vi "Func-엑셀 데이터를 그래프로 출력.vi"() -> ()   [LabVIEW 2015] (continued)
57.566\n45\t44.56\t57.56\n45\t44.56\t57.556\n45\t44.56\t57.547\n45\t44.56\t57.539\n45\t44.57\t57.535\n45\t44.57\t57.527\n45\t44.57\t57.522\n45\t44.58\t57.516\n45\t44.58\t57.513\n45\t44.58\t57.505\n45\t44.59\t57.495\n45\t44.59\t57.484\n45\t44.59\t57.475\n45\t44.59\t57.464\n45\t44.59\t57.451\n45\t44.6\t57.446\n45\t44.6\t57.445\n45\t44.6\t57.439\n45\t44.6\t57.435\n45\t44.61\t57.427\n45\t44.61\t57.424\n45\t44.61\t57.42\n45\t44.62\t57.407\n45\t44.62\t57.401\n45\t44.62\t57.397\n45\t44.62\t57.388\n45\t44.62\t57.386\n45\t44.63\t57.376\n45\t44.63\t57.366\n45\t44.64\t57.362\n45\t44.64\t57.358\n45\t44.64\t57.348\n45\t44.64\t57.339\n45\t44.64\t57.333\n45\t44.64\t57.33\n45\t44.64\t57.324\n45\t44.64\t57.311\n45\t44.65\t57.306\n45\t44.65\t57.302\n45\t44.66\t57.299\n45\t44.66\t57.284\n45\t44.67\t57.276\n45\t44.67\t57.272\n45\t44.67\t57.264\n45\t44.67\t57.255\n45\t44.68\t57.244\n45\t44.68\t57.24\n45\t44.68\t57.232\n45\t44.69\t57.225\n45\t44.69\t57.22\n45\t44.69\t57.216\n45\t44.7\t57.209\n45\t44.7\t57.203\n45\t44.7\t57.199\n45\t44.71\t57.189\n45\t44.71\t57.184\n45\t44.71\t57.18\n45\t44.71\t57.178\n45\t44.71\t57.173\n45\t44.72\t57.169\n45\t44.72\t57.159\n45\t44.73\t57.15\n45\t44.73\t57.139\n45\t44.73\t57.128\n45\t44.73\t57.12\n45\t44.73\t57.112\n45\t44.73\t57.105\n45\t44.73\t57.101\n45\t44.73\t57.097\n45\t44.74\t57.093\n45\t44.74\t57.086\n45\t44.74\t57.078\n45\t44.74\t57.073\n45\t44.75\t57.063\n45\t44.75\t57.056\n45\t44.75\t57.051\n45\t44.76\t57.048\n45\t44.76\t57.042\n45\t44.76\t57.037\n45\t44.77\t57.034\n45\t44.77\t57.025\n45\t44.77\t57.018\n45\t44.77\t57.013\n45\t44.77\t57.004\n45\t44.78\t56.999\n45\t44.78\t56.995\n45\t44.78\t56.989\n45\t44.78\t56.982\n45\t44.79\t56.973\n45\t44.8\t56.964\n45\t44.8\t56.957\n45\t44.8\t56.951\n45\t44.8\t56.937\n45\t44.8\t56.932\n45\t44.8\t56.927\n45\t44.8\t56.923\n45\t44.81\t56.917\n45\t44.81\t56.909\n45\t44.81\t56.902\n45\t44.81\t56.896\n45\t44.81\t56.886\n45\t44.81\t56.883\n45\t44.82\t56.88\n45\t44.82\t56.87\n45\t44.82\t56.866\n45\t44.82\t56.86\n45\t44.82\t56.854\n45\t44.82\t56.845\n45\t44.82\t56.835\n45\t44.82\t56.832\n45\t44.83\t56.829\n45\t44.83\t56.824\n45\t44.83\t56.816\n45\t44.83\t56.81\n45\t44.83\t56.807\n45\t44.83\t56.798\n45\t44.83\t56.794\n45\t44.83\t56.787\n45\t44.83\t56.784\n45\t44.83\t56.78\n45\t44.84\t56.772\n45\t44.84\t56.769\n45\t44.83\t56.761\n45\t44.84\t56.754\n45\t44.84\t56.744\n45\t44.84\t56.738\n45\t44.84\t56.735\n45\t44.84\t56.725\n45\t44.84\t56.724\n45\t44.84\t56.724\n45\t44.84\t56.716\n45\t44.85\t56.711\n45\t44.86\t56.698\n45\t44.87\t56.699\n45\t44.88\t56.693\n45\t44.89\t56.681\n45\t44.9\t56.676\n45\t44.91\t56.669\n45\t44.92\t56.659\n45\t44.93\t56.65\n45\t44.94\t56.642\n45\t44.95\t56.632\n45\t44.96\t56.629\n45\t44.97\t56.626\n45\t44.98\t56.623\n45\t45\t56.616\n45\t44.96\t56.611\n45\t44.96\t56.606\n45\t44.96\t56.6\n45\t44.96\t56.593\n45\t44.96\t56.581\n45\t44.96\t56.576\n45\t44.96\t56.566\n45\t44.96\t56.561\n45\t44.96\t56.555\n45\t44.96\t56.548\n45\t44.96\t56.547\n45\t44.96\t56.542\n45\t44.96\t56.539\n45\t44.96\t56.531\n45\t44.96\t56.526\n45\t44.96\t56.519\n45\t44.96\t56.513\n45\t44.96\t56.51\n45\t44.96\t56.502\n45\t44.96\t56.5\n45\t44.96\t56.493\n45\t44.96\t56.485\n45\t44.97\t56.48\n45\t44.97\t56.47\n45\t44.97\t56.461\n45\t44.97\t56.455\n45\t44.97\t56.449\n45\t44.97\t56.444\n45\t44.97\t56.437\n45\t44.97\t56.435\n45\t44.97\t56.428\n45\t44.97\t56.423\n45\t44.97\t56.418\n45\t44.97\t56.412\n45\t44.97\t56.411\n45\t44.97\t56.403\n45\t44.97\t56.399\n45\t44.97\t56.389\n45\t44.97\t56.383\n45\t44.97\t56.38\n45\t44.97\t56.372\n45\t44.97\t56.367\n45\t44.97\t56.362\n45\t44.97\t56.36\n45\t44.97\t56.353\n45\t44.97\t56.345\n45\t44.97\t56.34\n45\t44.97\t56.333\n45\t44.97\t56.327\n45\t44.97\t56.323\n45\t44.97\t56.317\n45\t44.97\t56.311\n45\t44.97\t56.304\n45\t44.97\t56.297\n45\t44.97\t56.291\n45\t44.97\t56.286\n45\t44.98\t56.278\n45\t44.98\t56.276\n45\t44.97\t56.275\n45\t44.97\t56.268\n45\t44.97\t56.264\n45\t44.97\t56.261\n45\t44.98\t56.26\n45\t44.98\t56.256\n45\t44.98\t56.25\n45\t44.98\t56.243\n45\t44.98\t56.239\n45\t44.98\t56.227\n45\t44.98\t56.216\n45\t44.98\t56.207\n45\t44.98\t56.203\n45\t44.98\t56.198\n45\t44.98\t56.192\n45\t44.98\t56.183\n45\t44.98\t56.18\n45\t44.98\t56.175\n45\t44.98\t56.167\n45\t44.98\t56.161\n45\t44.98\t56.16\n45\t44.98\t56.156\n45\t44.98\t56.154\n45\t44.98\t56.147\n45\t44.98\t56.138\n45\t44.98\t56.136\n45\t44.98\t56.125\n45\t44.98\t56.121\n45\t44.98\t56.113\n45\t44.98\t56.107\n45\t44.98\t56.104\n45\t44.98\t56.101\n45\t44.98\t56.092\n45\t44.98\t56.088\n45\t44.98\t56.082\n45\t44.98\t56.08\n45\t44.98\t56.076\n45\t44.98\t56.068\n45\t44.98\t56.066\n45\t44.98\t56.06\n45\t44.98\t56.06\n45\t44.98\t56.055\n45\t44.98\t56.047\n45\t44.98\t56.045\n45\t44.98\t56.035\n45\t44.98\t56.031\n45\t44.98\t56.025\n45\t44.98\t56.019\n45\t44.98\t56.018\n45\t44.98\t56.015\n45\t44.98\t56.007\n45\t45\t56.003\n45\t45\t55.997\n45\t45\t55.987\n45\t45\t55.978\n45\t45\t55.97\n45\t45\t55.969\n45\t45\t55.966\n45\t45\t55.962\n45\t45\t55.956\n45\t45\t55.954\n45\t45\t55.944\n45\t45\t55.941\n45\t45\t55.932\n45\t45\t55.924\n45\t45\t55.92\n45\t45\t55.916\n45\t45\t55.912\n45\t45\t55.907\n45\t45\t55.903\n45\t45\t55.895\n45\t45\t55.89\n45\t45\t55.884\n45\t44.98\t55.875\n45\t44.98\t55.868\n45\t45\t55.866\n45\t45\t55.862\n45\t45\t55.86\n45\t45\t55.857\n45\t44.98\t55.85\n45\t44.98\t55.849\n45\t44.98\t55.842\n45\t44.98\t55.834\n45\t44.98\t55.828\n45\t44.98\t55.823\n45\t44.98\t55.817\n45\t44.98\t55.811\n45\t44.98\t55.805\n45\t44.98\t55.801\n45\t44.98\t55.797\n45\t44.98\t55.787\n45\t44.98\t55.787\n45\t44.98\t55.782\n45\t44.98\t55.777\n45\t44.98\t55.772\n45\t44.98\t55.768\n45\t44.98\t55.762\n45\t44.98\t55.758\n45\t44.98\t55.755\n45\t44.98\t55.75\n45\t44.98\t55.745\n45\t44.98\t55.742\n45\t44.98\t55.736\n45\t44.98\t55.731\n45\t44.98\t55.727\n45\t44.98\t55.727\n45\t44.98\t55.72\n45\t44.98\t55.716\n45\t44.98\t55.713\n45\t45\t55.708\n45\t45\t55.698\n45\t44.98\t55.693\n45\t44.98\t55.69\n45\t45\t55.682\n45\t45\t55.681\n45\t45\t55.675\n45\t45\t55.671\n45\t45\t55.664\n45\t45\t55.661\n45\t45\t55.659\n45\t45\t55.652\n45\t45\t55.649\n45\t45\t55.643\n45\t45\t55.639\n45\t45\t55.631\n45\t45\t55.621\n45\t45\t55.618\n45\t45\t55.61\n45\t45\t55.607\n45\t45\t55.604\n45\t45\t55.602\n45\t45\t55.597\n45\t45\t55.589\n45\t45\t55.587\n45\t45\t55.581\n45\t45\t55.576\n45\t45\t55.575\n45\t45\t55.573\n45\t45\t55.571\n45\t45\t55.569\n45\t45\t55.557\n45\t45\t55.553\n45\t45\t55.543\n45\t45\t55.534\n45\t45\t55.53\n45\t45\t55.523\n45\t45\t55.521\n45\t45\t55.518\n45\t45\t55.511\n45\t45\t55.508\n45\t45\t55.502\n45\t45\t55.498\n45\t45\t55.494\n45\t45\t55.489\n45\t45\t55.486\n45\t45\t55.48\n45\t45\t55.475\n45\t45\t55.465\n45\t45\t55.46\n45\t45\t55.455\n45\t45\t55.449\n45\t45\t55.448\n45\t45\t55.445\n45\t45\t55.439\n45\t45\t55.436\n45\t45\t55.435\n45\t45\t55.429\n45\t45\t55.425\n45\t45\t55.42\n45\t45\t55.418\n45\t45\t55.416\n45\t45\t55.411\n45\t45\t55.406\n45\t45\t55.401\n45\t45\t55.391\n45\t45\t55.386\n45\t45\t55.381\n45\t45\t55.369\n45\t45\t55.368\n45\t45\t55.365\n45\t45\t55.365\n45\t45\t55.362\n45\t45\t55.357\n45\t45\t55.359\n45\t45\t55.354\n45\t45\t55.348\n45\t45\t55.344\n45\t45\t55.339\n45\t45\t55.333\n45\t45\t55.325\n45\t45\t55.323\n45\t45\t55.319\n45\t44.98\t55.312\n45\t44.98\t55.312\n45\t44.98\t55.309\n45\t44.98\t55.307\n45\t44.98\t55.299\n45\t44.98\t55.292\n45\t44.98\t55.287\n45\t44.98\t55.281\n45\t45\t55.277\n45\t45\t55.271\n45\t45\t55.268\n45\t44.98\t55.264\n45\t44.98\t55.259\n45\t44.98\t55.256\n45\t44.98\t55.247\n45\t44.98\t55.243\n45\t44.98\t55.24\n45\t44.98\t55.237\n45\t45\t55.235\n45\t45\t55.228\n45\t45\t55.225\n45\t45\t55.222\n45\t45\t55.219\n45\t45\t55.214\n45\t45\t55.212\n45\t45\t55.209\n45\t45\t55.204\n45\t45\t55.2\n45\t45\t55.196\n45\t45\t55.194\n45\t45\t55.194\n45\t45\t55.191\n45\t45\t55.186\n45\t45\t55.182\n45\t45\t55.178\n45\t45\t55.171\n45\t45\t55.162\n45\t45\t55.157\n45\t45\t55.155\n45\t45\t55.153\n45\t45\t55.147\n45\t45\t55.142\n45\t45\t55.139\n45\t45\t55.133\n45\t45\t55.129\n45\t45\t55.124\n45\t45\t55.117\n45\t45\t55.113\n45\t45\t55.109\n45\t45\t55.106\n45\t45\t55.102\n45\t45\t55.099\n45\t45\t55.093\n45\t45\t55.089\n45\t45\t55.086\n45\t45\t55.08\n45\t45\t55.076\n45\t45\t55.07\n45\t45\t55.066\n45\t45\t55.064\n45\t45\t55.06\n45\t45\t55.054\n45\t45\t55.046\n45\t45\t55.041\n45\t45\t55.039\n45\t45\t55.035\n45\t45\t55.026\n45\t45\t55.023\n45\t45\t55.023\n45\t45\t55.019\n45\t45\t55.016\n45\t45\t55.013\n45\t45\t55.013\n45\t45\t55.011\n45\t45\t55.009\n45\t45\t55.003\n45\t45\t54.998\n45\t45\t54.993\n45\t45\t54.986\n45\t45\t54.98\n45\t45\t54.977\n45\t45\t54.97\n45\t45\t54.966\n45\t45\t54.963\n45\t45\t54.964\n45\t45\t54.96\n45\t45\t54.954\n45\t45\t54.956\n45\t45\t54.953\n45\t45\t54.948\n45\t45\t54.942\n45\t45\t54.937\n45\t45\t54.935\n45\t45\t54.93\n45\t45\t54.925\n45\t45\t54.924\n45\t45\t54.918\n45\t45\t54.916\n45\t45\t54.909\n45\t45\t54.904\n45\t45\t54.902\n45\t45\t54.896\n45\t45\t54.893\n45\t45\t54.887\n45\t45\t54.887\n45\t45\t54.883\n45\t45\t54.878\n45\t45\t54.873\n45\t45\t54.868\n45\t45\t54.869\n45\t45\t54.865\n45\t45\t54.864\n45\t45\t54.861\n45\t45\t54.859\n45\t45\t54.857\n45\t45\t54.847\n45\t45\t54.842\n45\t45\t54.836\n45\t45\t54.836\n45\t45\t54.833\n45\t45\t54.829\n45\t45\t54.829\n45\t45\t54.826\n45\t45\t54.823\n45\t45\t54.809\n45\t45\t54.809\n45\t45\t54.805\n45\t45\t54.8\n45\t45\t54.798\n45\t45\t54.795\n45\t45\t54.797\n45\t45\t54.791\n45\t45\t54.788\n45\t45\t54.78\n45\t45\t54.778\n45\t45\t54.774\n45\t45\t54.764\n45\t45\t54.76\n45\t45\t54.755\n45\t45\t54.75\n45\t45\t54.743\n45\t45\t54.735\n45\t45\t54.734\n45\t45\t54.732\n45\t45\t54.732\n45\t45\t54.728\n45\t45\t54.725\n45\t45\t54.725\n45\t45\t54.722\n45\t45\t54.716\n45\t45\t54.713\n45\t45\t54.711\n45\t45\t54.711\n45\t45\t54.702\n45\t45\t54.698\n45\t45\t54.696\n45\t45\t54.689\n45\t45\t54.685\n45\t45\t54.681\n45\t45\t54.677\n45\t45\t54.676\n45\t45\t54.674\n45\t45\t54.67\n45\t45\t54.669\n45\t45\t54.664\n45\t45\t54.66\n45\t45\t54.655\n45\t45\t54.653\n45\t45\t54.649\n45\t45\t54.644\n45\t45\t54.642\n45\t45\t54.641\n45\t45\t54.636\n45\t45\t54.631\n45\t45\t54.623\n45\t45\t54.617\n45\t45\t54.617\n45\t45\t54.614\n45\t45\t54.613\n45\t45\t54.609\n45\t45\t54.605\n45\t45\t54.605\n45\t45\t54.596\n45\t45\t54.593\n45\t45\t54.591\n45\t45\t54.585\n45\t45\t54.586\n45\t45\t54.582\n45\t45\t54.58\n45\t45\t54.577\n45\t45\t54.57\n45\t45\t54.57\n45\t45\t54.563\n45\t45\t54.563\n45\t45\t54.555\n45\t45\t54.548\n45\t45\t54.545\n45\t45\t54.54\n45\t45\t54.537\n45\t45\t54.531\n45\t45\t54.527\n45\t45\t54.529\n45\t45\t54.529\n45\t45\t54.524\n45\t45\t54.523\n45\t45\t54.52\n45\t45\t54.521\n45\t45\t54.516\n45\t45\t54.509\n45\t45\t54.508\n45\t45\t54.505\n45\t45\t54.501\n45\t45\t54.497\n45\t45\t54.494\n45\t45\t54.493\n45\t45\t54.489\n45\t45\t54.487\n45\t45\t54.484\n45\t45\t54.479\n45\t45\t54.476\n45\t45\t54.473\n45\t45\t54.474\n45\t45\t54.47\n45\t45\t54.463\n45\t45\t54.461\n45\t45\t54.462\n45\t45\t54.456\n45\t45\t54.451\n45\t45\t54.448\n45\t45\t54.446\n45\t45\t54.444\n45\t45\t54.437\n45\t45\t54.437\n45\t45\t54.432\n45\t45\t54.426\n45\t45\t54.421\n45\t45\t54.415\n45\t45\t54.413\n45\t45\t54.408\n45\t45\t54.405\n45\t45\t54.403\n45\t45\t54.402\n45\t45\t54.399\n45\t45\t54.396\n45\t45\t54.393\n45\t45\t54.392\n45\t45\t54.39\n45\t45\t54.389\n45\t45\t54.384\n45\t45\t54.378\n45\t45\t54.377\n45\t45\t54.371\n45\t45\t54.367\n45\t45\t54.364\n45\t45\t54.364\n45\t45\t54.357\n45\t45\t54.353\n45\t45\t54.349\n45\t45\t54.346\n45\t45\t54.344\n45\t45\t54.339\n45\t45\t54.341\n45\t45\t54.339\n45\t45\t54.337\n45\t45\t54.329\n45\t45\t54.327\n45\t45\t54.324\n45\t45\t54.319\n45\t45\t54.317\n45\t45\t54.314\n45\t45\t54.317\n45\t45\t54.314\n45\t45\t54.311\n45\t45\t54.309\n45\t45\t54.303\n45\t45\t54.3\n45\t45\t54.295\n45\t45\t54.292\n45\t45\t54.286\n45\t45\t54.282\n45\t45\t54.278\n45\t45\t54.275\n45\t45\t54.27\n45\t45\t54.263\n45\t45\t54.259\n45\t45\t54.257\n45\t45\t54.255\n45\t45\t54.25\n45\t45\t54.248\n45\t45\t54.246\n45\t45\t54.245\n45\t45\t54.241\n45\t45\t54.237\n45\t45\t54.236\n45\t45\t54.233\n45\t45\t54.229\n45\t45\t54.224\n45\t45\t54.225\n45\t45\t54.223\n45\t45\t54.221\n45\t45\t54.218\n45\t45\t54.216\n45\t45\t54.214\n45\t45\t54.208\n45\t45\t54.202\n45\t45\t54.199\n45\t45\t54.199\n45\t45\t54.195\n45\t45\t54.195\n45\t45\t54.186\n45\t45\t54.185\n45\t45\t54.183\n45\t45\t54.176\n45\t45\t54.173\n45\t45\t54.167\n45\t45\t54.173\n45\t45\t54.168\n45\t45\t54.166\n45\t45\t54.166\n45\t45\t54.165\n45\t45\t54.166\n45\t45\t54.158\n45\t45\t54.157\n45\t45\t54.158\n45\t45\t54.152\n45\t45\t54.149\n45\t45\t54.143\n45\t45\t54.142\n45\t45\t54.14\n45\t45\t54.138\n45\t45\t54.133\n45\t45\t54.133\n45\t45\t54.134\n45\t45\t54.131\n45\t45\t54.129\n45\t45\t54.118\n45\t45\t54.117\n45\t45\t54.113\n45\t45\t54.107\n45\t45\t54.103\n45\t45\t54.098\n45\t45\t54.095\n45\t45\t54.092\n45\t45\t54.086\n45\t45\t54.085\n45\t45\t54.087\n45\t45\t54.085\n45\t45\t54.086\n45\t45\t54.085\n45\t45\t54.086\n45\t45\t54.084\n45\t45\t54.077\n45\t45\t54.078\n45\t45\t54.072\n45\t45\t54.07\n45\t45\t54.062\n45\t45\t54.061\n45\t45\t54.06\n45\t45\t54.051\n45\t45\t54.051\n45\t45\t54.046\n45\t45\t54.04\n45\t45\t54.033\n45\t45\t54.032\n45\t45\t54.037\n45\t45\t54.033\n45\t45\t54.031\n45\t45\t54.03\n45\t45\t54.028\n45\t45\t54.024\n45\t45\t54.013\n45\t45\t54.013\n45\t45\t54.011\n45\t45\t54.009\n45\t45\t54.005\n45\t45\t54.003\n45\t45\t54.002\n45\t45\t53.997\n45\t45\t53.998\n45\t45\t53.993\n45\t45\t53.993\n45\t45\t53.986\n45\t45\t53.982\n45\t45\t53.982\n45\t45\t53.974\n45\t45\t53.975\n45\t45\t53.971\n45\t45\t53.972\n45\t45\t53.97\n45\t45\t53.966\n45\t45\t53.964\n45\t45\t53.96\n45\t45\t53.961\n45\t45\t53.956\n45\t45\t53.954\n45\t45\t53.949\n45\t45\t53.945\n45\t45\t53.943\n45\t45\t53.939\n45\t45\t53.934\n45\t45\t53.93\n45\t45\t53.926\n45\t45\t53.925\n45\t45\t53.923\n45\t45\t53.918\n45\t45\t53.918\n45\t45\t53.917\n45\t45\t53.913\n45\t45\t53.911\n45\t45\t53.911\n45\t45\t53.907\n45\t45\t53.907\n45\t45\t53.905\n45\t45\t53.903\n45\t45\t53.898\n45\t45\t53.893\n45\t45\t53.889\n45\t45\t53.884\n45\t45\t53.883\n45\t45\t53.883\n45\t45\t53.885\n45\t45\t53.883\n45\t45\t53.882\n45\t45\t53.882\n45\t45\t53.88\n45\t45\t53.877\n45\t45\t53.872\n45\t45\t53.868\n45\t45\t53.865\n45\t45\t53.861\n45\t45\t53.859\n45\t45\t53.856\n45\t45\t53.855\n45\t45\t53.852\n45\t45\t53.852\n45\t45\t53.846\n45\t45\t53.835\n45\t45\t53.834\n45\t45\t53.831\n45\t45\t53.829\n45\t45\t53.826\n45\t45\t53.829\n45\t45\t53.829\n45\t45\t53.826\n45\t45\t53.823\n45\t45\t53.82\n45\t45\t53.816\n45\t45\t53.815\n45\t45\t53.813\n45\t45\t53.808\n45\t45\t53.807\n45\t45\t53.805\n45\t45\t53.807\n45\t45\t53.803\n45\t45\t53.802\n45\t45\t53.804\n45\t45\t53.795\n45\t45\t53.794\n45\t45\t53.79\n45\t45\t53.787\n45\t45\t53.782\n45\t45\t53.775\n45\t45\t53.777\n45\t45\t53.775\n45\t45\t53.775\n45\t45\t53.773\n45\t45\t53.773\n45\t45\t53.775\n45\t45\t53.769\n45\t45\t53.763\n45\t45\t53.756\n45\t45\t53.754\n45\t45\t53.751\n45\t45\t53.745\n45\t45\t53.743\n45\t45\t53.745\n45\t45\t53.741\n45\t45\t53.739\n45\t45\t53.737\n45\t45\t53.735\n45\t45\t53.733\n45\t45\t53.73\n45\t45\t53.728\n45\t45\t53.726\n45\t45\t53.722\n45\t45\t53.721\n45\t45\t53.719\n45\t45\t53.716\n45\t45\t53.713\n45\t45\t53.714\n45\t45\t53.714\n45\t45\t53.714\n45\t45\t53.712\n45\t45\t53.709\n45\t45\t53.706\n45\t45\t53.7\n45\t45\t53.694\n45\t45\t53.691\n45\t45\t53.689\n45\t45\t53.687\n45\t45\t53.687\n45\t45\t53.683\n45\t45\t53.685\n45\t45\t53.678\n45\t45\t53.675\n45\t45\t53.67\n45\t45\t53.665\n45\t45\t53.668\n45\t45\t53.66\n45\t45\t53.659\n45\t45\t53.658\n45\t45\t53.66\n45\t45\t53.656\n45\t45\t53.653\n45\t45\t53.649\n45\t45\t53.646\n45\t45\t53.645\n45\t45\t53.64\n45\t45\t53.641\n45\t45\t53.635\n45\t45\t53.637\n45\t45\t53.638\n45\t45\t53.637\n45\t45\t53.633\n45\t45\t53.63\n45\t45\t53.63\n45\t45\t53.623\n45\t45\t53.622\n45\t45\t53.616\n45\t45\t53.618\n45\t45\t53.617\n45\t45\t53.611\n45\t45\t53.613\n45\t45\t53.609\n45\t45\t53.605\n45\t45\t53.601\n45\t45\t53.6\n45\t45\t53.6\n45\t45\t53.596\n45\t45\t53.595\n45\t45\t53.598\n45\t45\t53.596\n45\t45\t53.593\n45\t45\t53.589\n45\t45\t53.589\n45\t45\t53.584\n45\t45\t53.581\n45\t45\t53.577\n45\t45\t53.573\n45\t45\t53.571\n45\t45\t53.57\n45\t45\t53.569\n45\t45\t53.564\n45\t45\t53.563\n45\t45\t53.562\n45\t45\t53.561\n45\t45\t53.556\n45\t45\t53.555\n45\t45\t53.555\n45\t45\t53.551\n45\t45\t53.546\n45\t45\t53.541\n45\t45\t53.536\n45\t45\t53.531\n45\t45\t53.525\n45\t45\t53.528\n45\t45\t53.529\n45\t45\t53.528\n45\t45\t53.53\n45\t45\t53.527\n45\t45\t53.528\n45\t45\t53.524\n45\t45\t53.523\n45\t45\t53.521\n45\t45\t53.519\n45\t45\t53.518\n45\t45\t53.514\n45\t45\t53.511\n45\t45\t53.505\n45\t45\t53.501\n45\t45\t53.503\n45\t45\t53.5\n45\t45\t53.502\n45\t45\t53.5\n45\t45\t53.496\n45\t45\t53.493\n45\t45\t53.489\n45\t45\t53.487\n45\t45\t53.482\n45\t45\t53.482\n45\t45\t53.479\n45\t45\t53.479\n45\t45\t53.471\n45\t45\t53.468\n45\t45\t53.471\n45\t45\t53.464\n45\t45\t53.464\n45\t45\t53.462\n45\t45\t53.465\n45\t45\t53.465\n45\t45\t53.458\n45\t45\t53.458\n45\t45\t53.457\n45\t45\t53.455\n45\t45\t53.45\n45\t45\t53.446\n45\t45\t53.446\n45\t45\t53.444\n45\t45\t53.441\n45\t45\t53.439\n45\t45\t53.439\n45\t45\t53.441\n45\t45\t53.438\n45\t45\t53.436\n45\t45\t53.437\n45\t45\t53.437\n45\t45\t53.432\n45\t45\t53.432\n45\t45\t53.431\n45\t45\t53.431\n45\t45\t53.429\n45\t45\t53.427\n45\t45\t53.428\n45\t45\t53.422\n45\t45\t53.421\n45\t45\t53.418\n45\t45\t53.416\n45\t45\t53.413\n45\t45\t53.411\n45\t45\t53.405\n45\t45\t53.401\n45\t45\t53.401\n45\t45\t53.4\n45\t45\t53.399\n45\t45\t53.397\n45\t45\t53.397\n45\t45\t53.392\n45\t45\t53.389\n45\t45\t53.386\n45\t45\t53.382\n45\t45\t53.382\n45\t45\t53.375\n45\t45\t53.377\n45\t45\t53.373\n45\t45\t53.368\n45\t45\t53.368\n45\t45\t53.365\n45\t45\t53.364\n45\t45\t53.365\n45\t45\t53.363\n45\t45\t53.364\n45\t45\t53.359\n45\t45\t53.36\n45\t45\t53.36\n45\t45\t53.357\n45\t45\t53.354\n45\t45\t53.352\n45\t45\t53.355\n45\t45\t53.353\n45\t45\t53.352\n45\t45\t53.35\n45\t45\t53.348\n45\t45\t53.346\n45\t45\t53.344\n45\t45\t53.336\n45\t45\t53.333\n45\t45\t53.329\n45\t45\t53.33\n45\t45\t53.327\n45\t45\t53.324\n45\t45\t53.321\n45\t45\t53.319\n45\t45\t53.318\n45\t45\t53.314\n45\t45\t53.315\n45\t45\t53.312\n45\t45\t53.312\n45\t45\t53.312\n45\t45\t53.311\n45\t45\t53.309\n45\t45\t53.302\n45\t45\t53.301\n45\t45\t53.302\n45\t45\t53.299\n45\t45\t53.295\n45\t45\t53.293\n45\t45\t53.295\n45\t45\t53.292\n45\t45\t53.292\n45\t45\t53.293\n45\t45\t53.292\n45\t45\t53.292\n45\t45\t53.29\n45\t45\t53.293\n45\t45\t53.287\n45\t45\t53.283\n45\t45\t53.282\n45\t45\t53.277\n45\t45\t53.276\n45\t45\t53.273\n45\t45\t53.273\n45\t45\t53.269\n45\t45\t53.264\n45\t45\t53.265\n45\t45\t53.259\n45\t45\t53.256\n45\t45\t53.253\n45\t45\t53.249\n45\t45\t53.249\n45\t45\t53.245\n45\t45\t53.244\n45\t45\t53.243\n45\t45\t53.244\n45\t45\t53.244\n45\t45\t53.239\n45\t45\t53.238\n45\t45\t53.234\n45\t45\t53.233\n45\t45\t53.229\n45\t45\t53.23\n45\t45\t53.229\n45\t45\t53.232\n45\t45\t53.23\n45\t45\t53.227\n45\t45\t53.223\n45\t45\t53.221\n45\t45\t53.219\n45\t45\t53.219\n45\t45\t53.219\n45\t45\t53.218\n45\t45\t53.22\n45\t45\t53.216\n45\t45\t53.216\n45\t45\t53.21\n45\t45\t53.211\n45\t45\t53.209\n45\t45\t53.206\n45\t45\t53.207\n45\t45\t53.199\n45\t45\t53.2\n45\t45\t53.197\n45\t45\t53.195\n45\t45\t53.192\n45\t45\t53.189\n45\t45\t53.192\n45\t45\t53.187\n45\t45\t53.184\n45\t45\t53.183\n45\t45\t53.181\n45\t45\t53.183\n45\t45\t53.177\n45\t45\t53.177\n45\t45\t53.179\n45\t45\t53.175\n45\t45\t53.173\n45\t45\t53.169\n45\t45\t53.167\n45\t45\t53.168\n45\t45\t53.164\n45\t45\t53.161\n45\t45\t53.16\n45\t45\t53.159\n45\t45\t53.158\n45\t45\t53.155\n45\t45\t53.152\n45\t45\t53.151\n45\t45\t53.151\n45\t45\t53.149\n45\t45\t53.147\n45\t45\t53.143\n45\t45\t53.141\n45\t45\t53.139\n45\t45\t53.137\n45\t45\t53.136\n45\t45\t53.133\n45\t45\t53.135\n45\t45\t53.136\n45\t45\t53.133\n45\t45\t53.128\n45\t45\t53.125\n45\t45\t53.128\n45\t45\t53.127\n45\t45\t53.123\n45\t45\t53.123\n45\t45\t53.127\n45\t45\t53.129\n45\t45\t53.125\n45\t45\t53.124\n45\t45\t53.119\n45\t45\t53.118\n45\t45\t53.114\n45\t45\t53.111\n45\t45\t53.109\n45\t45\t53.107\n45\t45\t53.109\n45\t45\t53.11\n45\t45\t53.106\n45\t45\t53.104\n45\t45\t53.105\n45\t45\t53.098\n45\t45\t53.095\n45\t45\t53.088\n45\t45\t53.088\n45\t45\t53.086\n45\t45\t53.08\n
